vi "NotifierPartB.vi"() -> ()   [LabVIEW 2014]
panel:
  out "count":i32
  in  "stop":bool
  out "NumericOut":i32
  # "Part B"
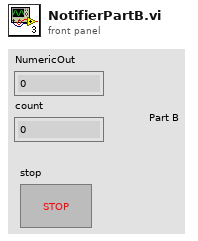
[diagram p1: front panel]
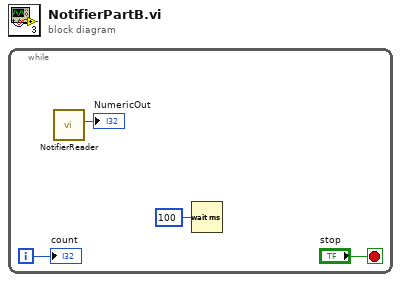
[diagram p0: block diagram]
diagram:
  n1 = while {
    i -> [w2]
    stop <- "stop" stop-if-true
    n2 = call "NotifierReader.vi"() -> ("NumericOut"=→"NumericOut":i32)  [unwired: 11 in]
    n3 = Wait (ms)(milliseconds to wait=u32 100) -> ()  [unwired: 1 out]
    "count" <- w2
  }
